vi "Between.vi"(9 "Hallway Position":i32, 10 "Room":string, 11 "Position":i32) -> (3 "Betwwen?":bool)   [LabVIEW 2019, in "23.lvlib"]
uses:
  23.lvlib
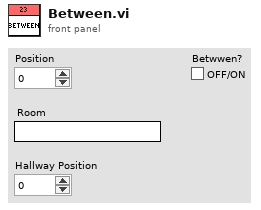
[diagram p1: front panel]
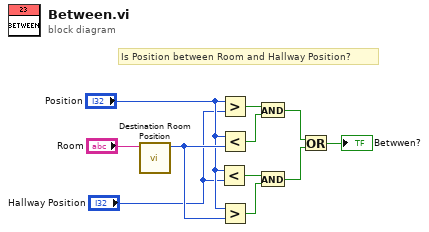
[diagram p0: block diagram]
diagram:
  # "Is Position between Room and Hallway Position?"
  n1 = call "Destination Room Position.vi"("Amphipod Type"="Room") -> ("Destination Room Position"=w6:i32)  [unwired: 10 in]
  n2 = Less?(x="Position", y="Hallway Position") -> (x < y?=w2:bool)
  n3 = Greater?(x="Position", y="Hallway Position") -> (0:w7:bool)
  n4 = Less?(x="Position", y=w6) -> (x < y?=w8:bool)
  n5 = Greater?(x="Position", y=w6) -> (0:w3:bool)
  n6 = And(x=w7, y=w8) -> (x .and. y?=w9:bool)
  n7 = And(x=w2, y=w3) -> (x .and. y?=w10:bool)
  n8 = Or(x=w9, y=w10) -> (x .or. y?=→"Betwwen?":bool)
